vi "解析命令.vi"(5 "Robot Status 2":string="<ToPC><ToX>345.114777</ToX></ToPC><ToPC><ToY>400.628418</ToY></ToPC><ToPC><ToA>-90.3234</ToA></ToPC>") -> (0 "C":dbl, 1 "y":dbl, 2 "x":dbl)   [LabVIEW 2016]
panel:
  out "C":string
  out "Y":string
  out "X":string
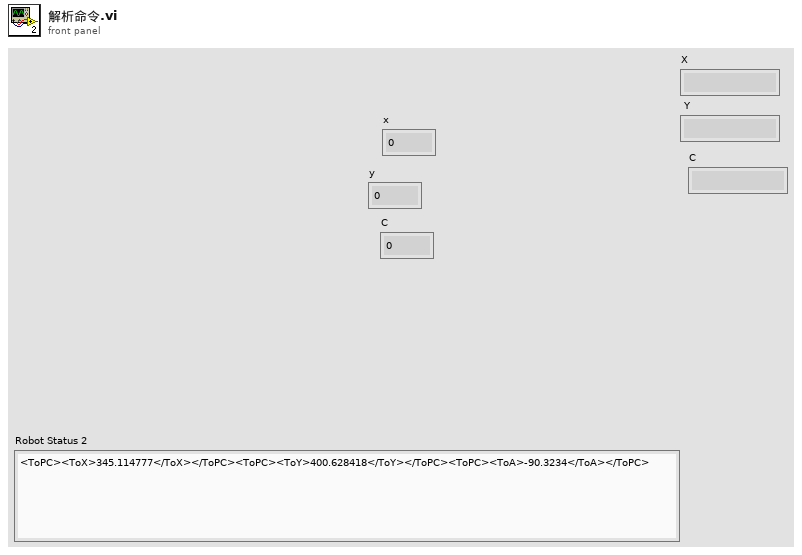
[diagram p1: front panel]
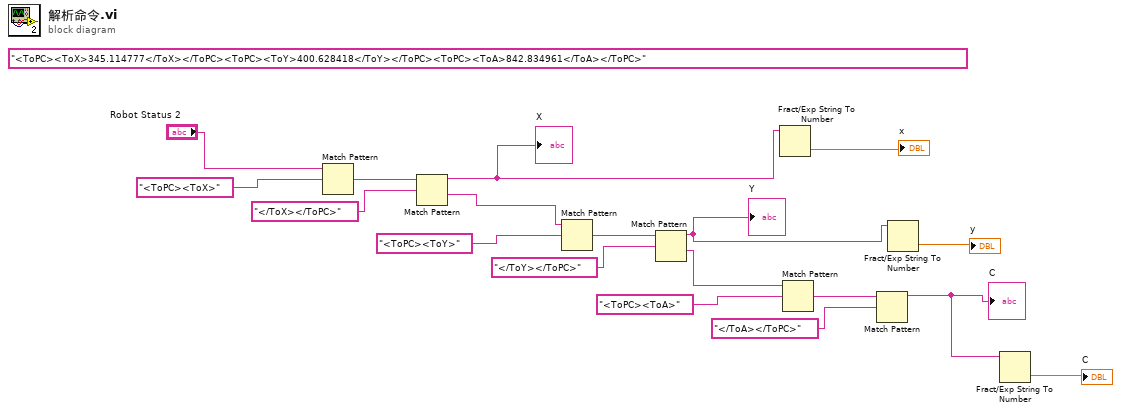
[diagram p0: block diagram]
diagram:
  (unwired) "<ToPC><ToX>345.114777</ToX></ToPC><ToPC><ToY>400.628418</ToY></ToPC><ToPC><ToA>842.834961</ToA></ToPC>"
  n1 = Match Pattern(string="Robot Status 2", regular expression="<ToPC><ToX>" ("正则表达式")) -> (after substring=w16:string)  [unwired: 1 in, 3 out]
  n2 = Match Pattern(string=w16, regular expression="</ToX></ToPC>" ("正则表达式")) -> (before substring=w9:string, after substring=w10:string)  [unwired: 1 in, 2 out]
  "X" <- w9
  n3 = Match Pattern(string=w10, regular expression="<ToPC><ToY>" ("正则表达式")) -> (after substring=w11:string)  [unwired: 1 in, 3 out]
  n4 = Match Pattern(string=w11, regular expression="</ToY></ToPC>" ("正则表达式")) -> (before substring=w8:string, after substring=w3:string)  [unwired: 1 in, 2 out]
  "Y" <- w8
  n5 = Fract/Exp String To Number(string=w9) -> (number=→"x":dbl)  [unwired: 3 in, 1 out]
  n6 = Match Pattern(string=w3, regular expression="<ToPC><ToA>" ("正则表达式")) -> (after substring=w6:string)  [unwired: 1 in, 3 out]
  n7 = Match Pattern(string=w6, regular expression="</ToA></ToPC>" ("正则表达式")) -> (before substring=w1:string)  [unwired: 1 in, 3 out]
  "C" <- w1
  n8 = Fract/Exp String To Number(string=w8) -> (number=→"y":dbl)  [unwired: 3 in, 1 out]
  n9 = Fract/Exp String To Number(string=w1) -> (number=→"C":dbl)  [unwired: 3 in, 1 out]
